vi "Status.vi"(8 "error in (no error)":errorcluster, 11 "Integrator in":refnum<class "Integrator.lvclass">) -> (0 "error out":errorcluster, 2 "Integrating":bool, 3 "Integrator out":refnum<class "Integrator.lvclass">)   [LabVIEW 2016, in "Integrator.lvclass"]
uses:
  Integrator.lvclass
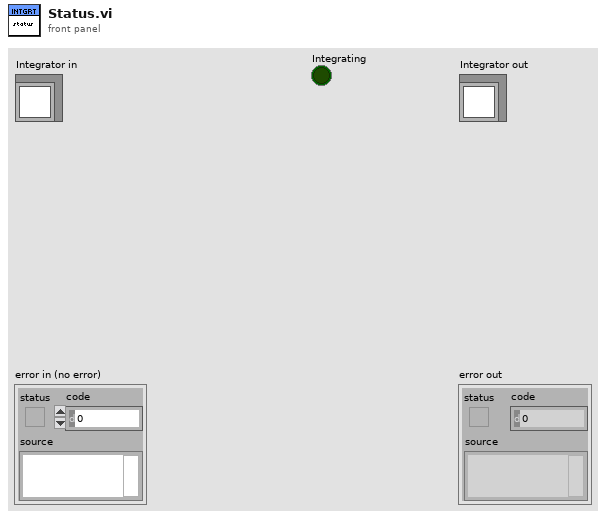
[diagram p1: front panel]
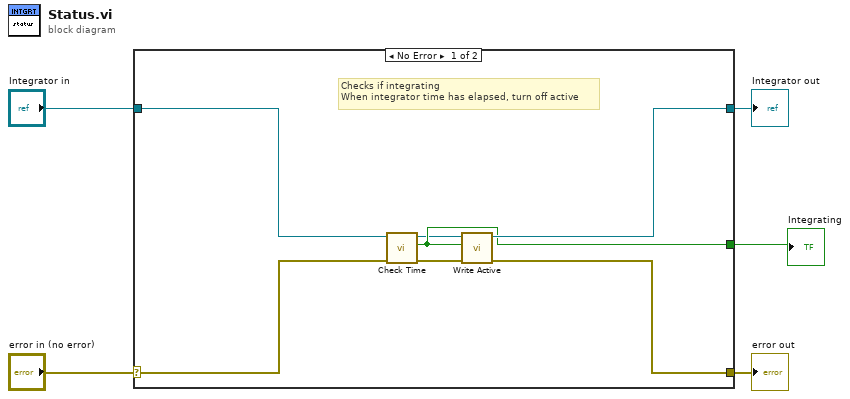
[diagram p0: block diagram]
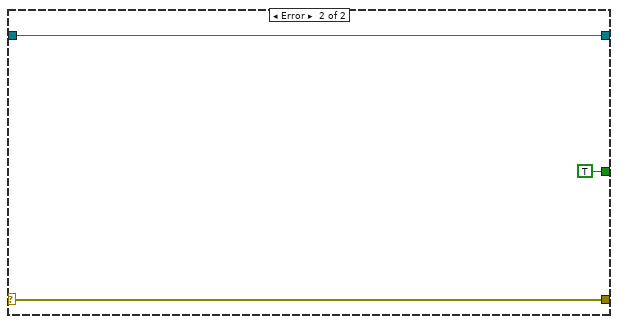
[diagram p2: hidden frame]
diagram:
  n1 = case shown="No Error" "error in (no error)" {
    selector: "error in (no error)" -> [w6 w15]
    tunnel: [w11 w15] -> w4
    tunnel: [w12 w14] -> w2
    tunnel: "Integrator in" -> [w7 w14]
    tunnel: [w10 TRUE ("Integrating")] -> w1
    frame No Error {
      # "Checks if integrating\nWhen integrator time has elapsed, turn off active"
      n2 = call-dynamic "Check Time.vi"("error in (no error)"=w6, "Integrator in"=w7) -> ("error out"=w9:errorcluster, "Integrating"=w10:bool, "Integrator out"=w8:refnum<class "Integrator.lvclass">)  [unwired: 7 in]
      n3 = call-dynamic "Write Active.vi"("error in (no error)"=w9, "Active"=w10, "Integrator in"=w8) -> ("error out"=w11:errorcluster, "Integrator out"=w12:refnum<class "Integrator.lvclass">)  [unwired: 7 in]
    }
    frame Error {
    }
  }
  "error out" <- w4
  "Integrator out" <- w2
  "Integrating" <- w1
